vi "Create_Raw_data_file.vi"(4 "No of averages":i32=1, 5 "End time":dbl, 6 "Start time":dbl, 7 "Setup filename":string) -> (0 "Error String":string, 1 "Values":string[][](array[string]), 2 "Header Comments":string[](array[string]), 3 "Column headers":string[](array[string]))   [LabVIEW 2017]
uses:
  File/Setup_Filetype.ctl
  Controls/Post_Process.ctl
  Globals/Preference_global.vi
  Globals/Meas_global.vi
  Globals/Trav_pos_global.vi
  Globals/Constants_global.vi
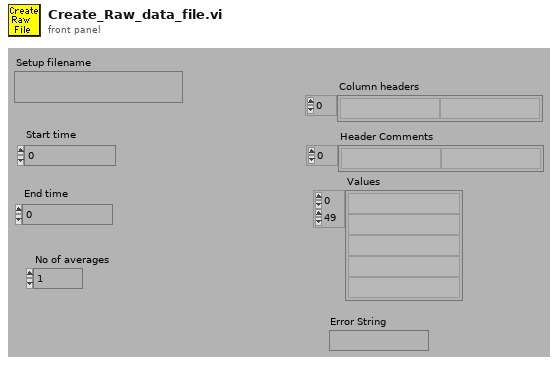
[diagram p1: front panel]
types:
  T1 = typedef "Post_Process.ctl" = enum16{"Take New Data", "Post Process Raw Data File"}
  T2 = typedef "Server_Comms.ctl" = enum16{"Server Link Healthy", "Do Not Link To Server"}
  T3 = typedef "Setup_Filetype.ctl" = enum16{"Measurement Setups", "Calibration Setups", "General", "Results File Plotter Setups", "Speed Calib Tweaks"}
  T4 = typedef "Traverse_cluster.ctl" = cluster{"Start X":sgl, "Start Y":sgl, "Start Z":sgl, "End X":sgl, "End Y":sgl, "End Z":sgl, "No. of pts.":i32, "Spacing":T5, "Filename":path, "Tunnel Speed":dbl, "Averaging time (min)":dbl, "Extra Commands":string, "Carrier_1 Q (l/min)":dbl, "Carrier_2 Q (l/min)":dbl, "Trace Gas Concentration (%)":dbl, "Specific Arguments":string, "Comments":string, "Row No":i32, "Row Type Selector":T6, "Completion time":string, "Row Duration (mins)":dbl, "No. of Valid pts.":i32, "Meas Setup File":string}
  T5 = typedef "Spacing.ctl" = enum16{"Linear", "Log", "Gauss", "Specified", "N/A"}
  T6 = typedef "Multi_run_mode.ctl" = enum16{"Move Traverse Only", "Set Tunnel Speed Only", "Set Source Only", "Set Measurement Conditions", "Single Measurement", "Vertical Profile", "Lateral Profile", "Longitudinal Profile", "Explore Volume", "Multi-Axis Profile", "Auto Calibrate", "Meas Fast FID Bkgnd", "Check Beam Power", "Scanning Valve Measurement", "Run VI Named:", "Set ADAM Ch", "Wait (minutes)", "Send Message", "Synchronize With:", "Fall Back to this Row", "Turn Off Row Repeating", "Blank Row", "Traverse 3D Volume"}
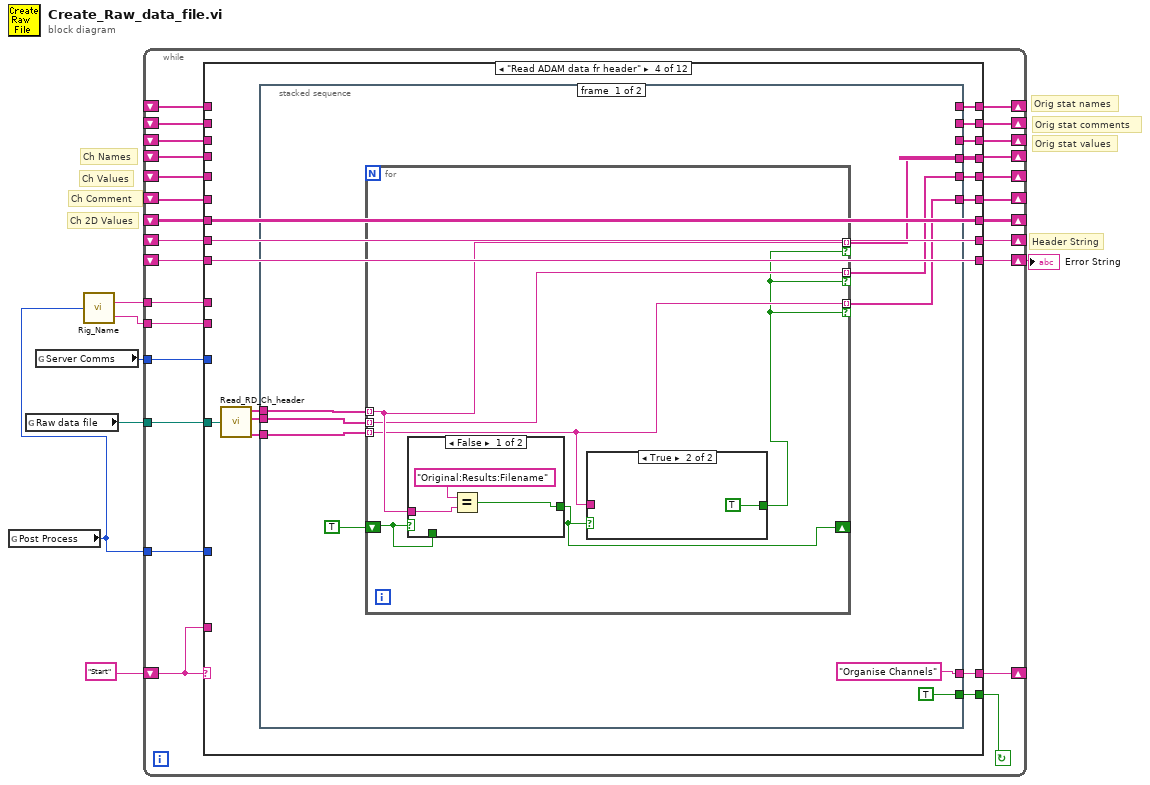
[diagram p0: block diagram]
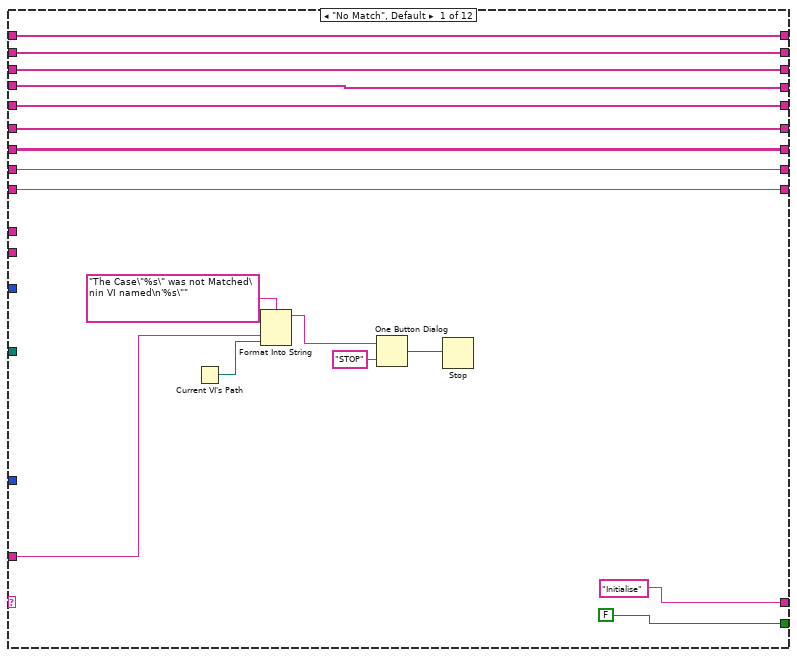
[diagram p2: hidden frame]
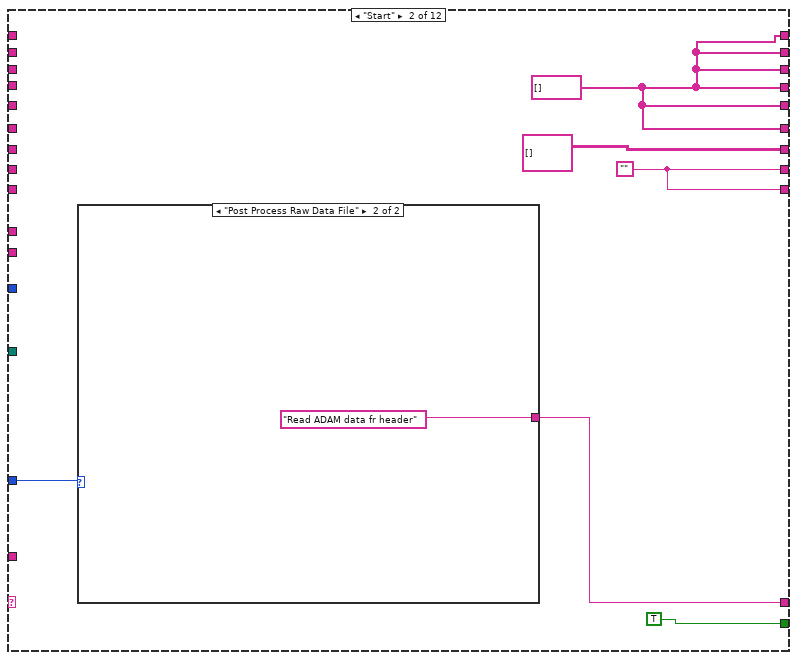
[diagram p3: hidden frame]
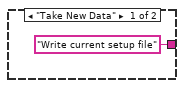
[diagram p4: hidden frame]
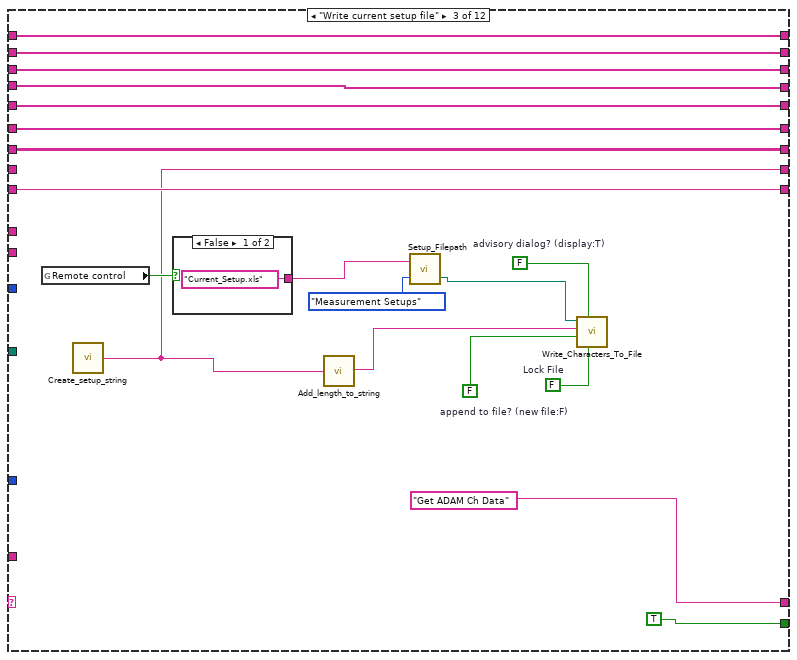
[diagram p5: hidden frame]
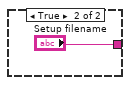
[diagram p6: hidden frame]
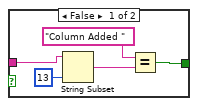
[diagram p7: hidden frame]
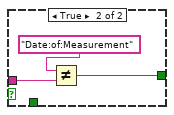
[diagram p8: hidden frame]
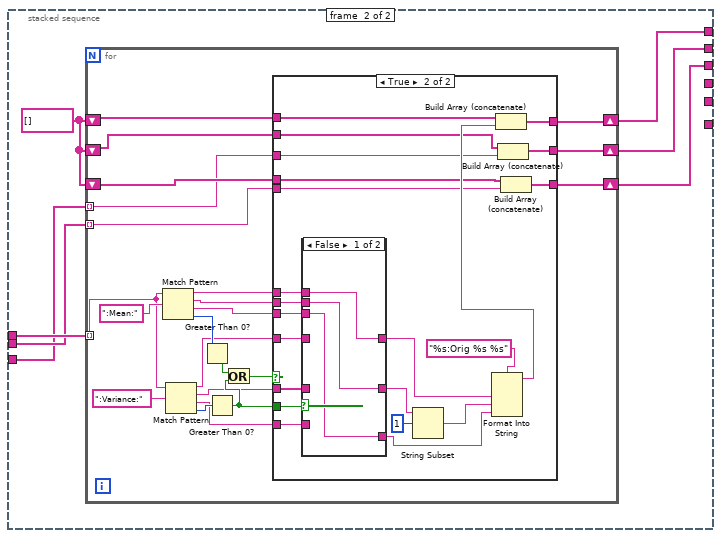
[diagram p9: hidden frame]
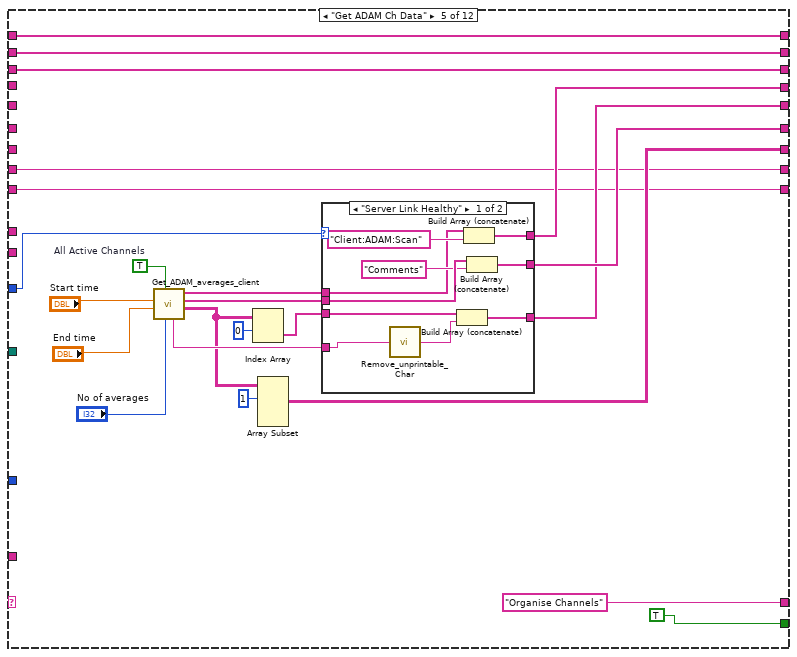
[diagram p12: hidden frame]
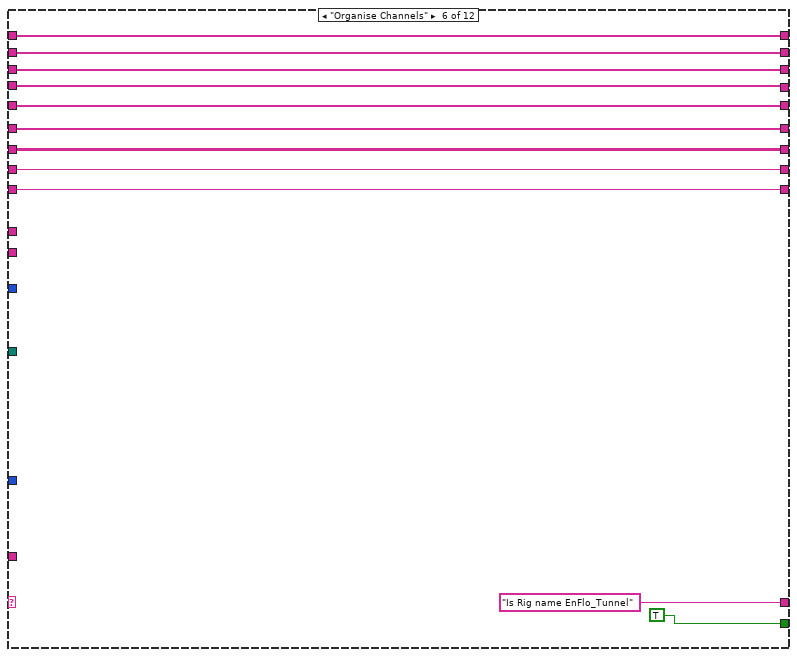
[diagram p14: hidden frame]
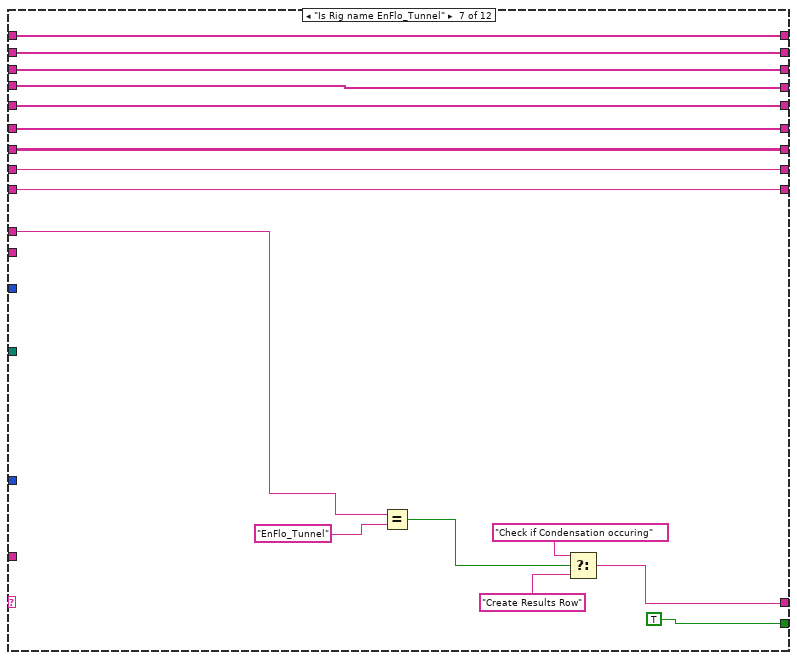
[diagram p15: hidden frame]
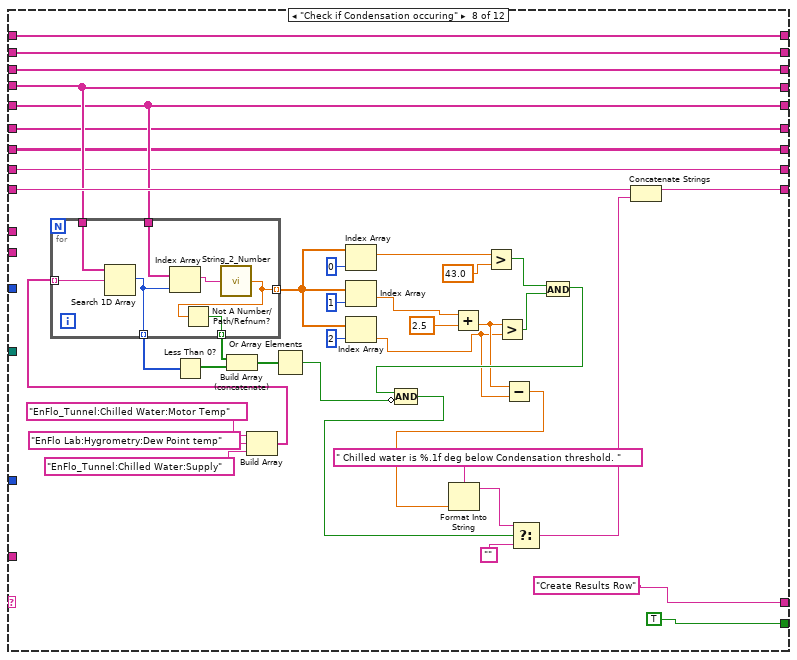
[diagram p16: hidden frame]
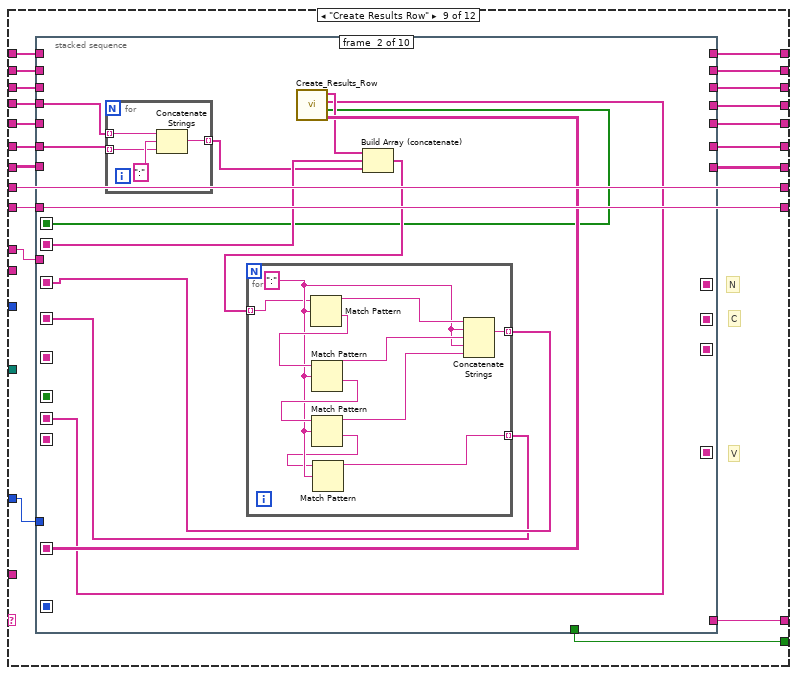
[diagram p17: hidden frame]
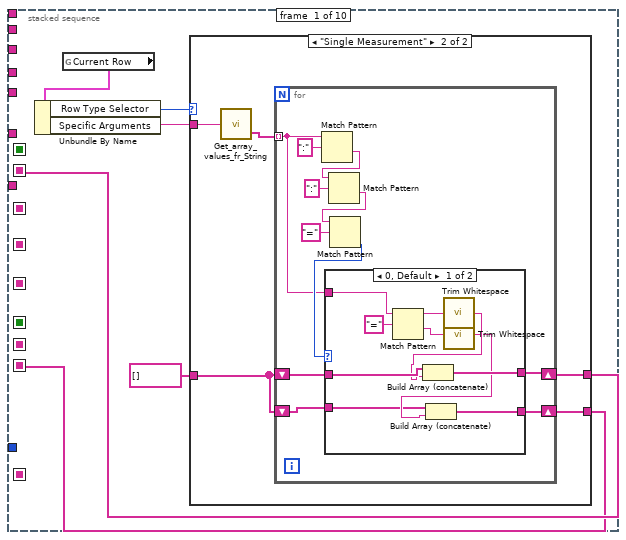
[diagram p18: hidden frame]
diagram:
  # "Orig stat values"
  # "Orig stat comments"
  # "Orig stat names"
  # "Header String"
  # "Ch 2D Values"
  # "Ch Comment"
  # "Ch Values"
  # "Ch Names"
  n1 = global read "Meas_global.vi" "Post Process"() -> (w3:T1)
  n2 = global read "Meas_global.vi" "Raw data file"() -> (w6:path)
  n3 = global read "Preference_global.vi" "Server Comms"() -> (w5:T2)
  n4 = call "Rig_Name.vi"("Post Process"=w3) -> ("Rig Setup before dash"=w2:string, "Hard Disk name"=w1:string)
  n5 = while {
    tunnel: w5 -> [w16]
    tunnel: w6 -> [w17]
    tunnel: w3 -> [w18]
    shift-left: _ -> [w20]
    shift-right: [w19] -> _
    shift-left: _ -> [w26]
    shift-right: [w25] -> w4
    shift-left: _ -> [w21]
    shift-right: [w27] -> _
    shift-left: _ -> [w22]
    shift-right: [w29] -> _
    shift-left: _ -> [w23]
    shift-right: [w28] -> _
    shift-left: _ -> [w24]
    shift-right: [w30] -> _
    shift-left: "Start" -> [w31]
    shift-right: [w32] -> _
    tunnel: w2 -> [w15]
    tunnel: w1 -> [w14]
    shift-right: [w10] -> _
    shift-left: _ -> [w11]
    shift-right: [w8] -> _
    shift-left: _ -> [w9]
    shift-right: [w12] -> _
    shift-left: _ -> [w13]
    stop <- w33 continue-if-true
    n6 = case shown="\"Read ADAM data fr header\"" w31 {
      tunnel: [FALSE TRUE TRUE w83 TRUE TRUE TRUE TRUE w299 TRUE TRUE FALSE] -> w33
      tunnel: ["Initialise" w52 "Get ADAM Ch Data" w94 "Organise Channels" "Is Rig name EnFlo_Tunnel" w236 "Create Results Row" w311 "Add Raw Data header info" "Add Raw Data fr Tempory file" "End"] -> w32
      tunnel: w31 -> [w45 _ _ _ _ _ _ _ _ _ _ _]
      tunnel: [w42 w51 w77 w85 w192 w226 w244 w254 w308 w614 w644 w661] -> w30
      tunnel: [w40 w51 w75 w86 w191 w224 w242 w252 w305 w625 w646 w663] -> w29
      tunnel: [w41 w51 w76 w84 w190 w225 w243 w253 w301 w626 w645 w662] -> w28
      tunnel: [w39 string[][] [] w74 w92 w188 w223 w241 w251 w303 w617 w647 w664] -> w27
      tunnel: w26 -> [w38 _ w72 w93 w187 w221 w238 w257 w309 w630 w648 w665]
      tunnel: [w38 w54 w72 w93 w187 w221 w238 w255 w309 w630 w648 w665] -> w25
      tunnel: w24 -> [w42 _ w77 _ _ w226 w244 w254 w307 w614 w644 w661]
      tunnel: w23 -> [w41 _ w76 _ _ w225 w243 w253 w302 w626 w645 w662]
      tunnel: w22 -> [w40 _ w75 _ _ w224 w242 w252 w306 w625 w646 w663]
      tunnel: w21 -> [w39 _ w74 w92 _ w223 w241 w251 w304 w617 w647 w664]
      tunnel: w20 -> [w37 _ _ w91 w186 w222 w239 w249 w310 w619 w641 w660]
      tunnel: [w37 w54 w66 w91 w186 w222 w239 w249 w310 w622 w640 ""] -> w19
      tunnel: w18 -> [_ w53 _ _ _ _ _ _ w300 _ _ _]
      tunnel: w17 -> [_ _ _ w90 _ _ _ _ _ _ _ w656]
      tunnel: w16 -> [_ _ _ _ w185 _ _ _ _ _ _ _]
      tunnel: w15 -> [_ _ _ _ _ _ w233 _ w298 _ _ _]
      tunnel: w14 -> [_ _ _ _ _ _ _ _ _ _ _ _]
      tunnel: w13 -> [w36 _ w64 _ w184 w220 w231 w248 w296 w611 w639 w653]
      tunnel: [w36 w51 w64 w82 w184 w220 w231 w248 w297 w611 w639 w653] -> w12
      tunnel: w11 -> [w35 _ w63 _ w183 w219 w230 w247 w295 w610 w638 w652]
      tunnel: [w35 w51 w63 w81 w183 w219 w230 w247 w294 w610 w638 w652] -> w10
      tunnel: w9 -> [w34 _ w62 _ w182 w218 w229 w246 w292 w609 w637 w651]
      tunnel: [w34 w51 w62 w80 w182 w218 w229 w246 w293 w609 w637 w651] -> w8
      frame "No Match", Default {
        n7 = Current VI's Path() -> (path=w44:path)
        n8 = Format Into String(format string="The Case\"%s\" was not Matched\nin VI named\n'%s\"" ("Format String"), w45, w44) -> (resulting string=w48:string)  [unwired: 2 in, 1 out]
        n9 = One Button Dialog(message=w48, button name ("OK")="STOP") -> (true=w46:bool)
        n10 = Stop(stop? (T)=w46) -> ()
      }
      frame "Start" {
        w54 = ""
        w51 = string[] []
        n11 = case shown="\"Post Process Raw Data File\"" w53 {
          tunnel: ["Write current setup file" "Read ADAM data fr header"] -> w52
          frame "Take New Data" {
          }
          frame "Post Process Raw Data File" {
          }
        }
      }
      frame "Write current setup file" {
        w67 = FALSE  # Lock File
        w70 = FALSE  # advisory dialog? (display:T)
        w71 = FALSE  # append to file? (new file:F)
        n12 = global read "Meas_global.vi" "Remote control"() -> (w69:bool)
        n13 = call "Create_setup_string.vi"() -> ("Setup String"=w66:string)  [unwired: 1 out]
        n14 = case shown="False" w69 {
          tunnel: ["Current_Setup.xls" ("Setup filename") "Setup filename"] -> w60
          frame False {
          }
          frame True {
          }
        }
        n15 = call "Add_length_to_string.vi"("String in"=w66) -> ("String out"=w68:string)
        n16 = call "Setup_Filepath.vi"("Setup File Type"=Setup_Filetype."Measurement Setups", "Filename in"=w60) -> ("Filename Out"=w59:path)  [unwired: 1 out]
        n17 = call "Write_Characters_To_File.vi"("file path (dialog if empty)"=w59, "advisory dialog? (display:T)"=w70, "character string"=w68, "append to file? (new file:F)"=w71, "Lock File"=w67) -> ()  [unwired: 4 out]
      }
      frame "Read ADAM data fr header" {
        n18 = call "Read_RD_Ch_header.vi"("Raw data file"=w90) -> ("Ch Name Out"=w88:string[], "Ch Values"=w87:string[], "Comments"=w89:string[])  [unwired: 1 out]
        n19 = stacked-sequence {
          tunnel: ["Organise Channels" _] -> w94
          tunnel: w89 -> [w101 w125]
          tunnel: w88 -> [w100 w128]
          tunnel: w87 -> [w99 w126]
          tunnel: [w95 _] -> w86
          tunnel: [w97 _] -> w85
          tunnel: [w96 _] -> w84
          tunnel: [TRUE _] -> w83
          tunnel: [_ w124] -> w82
          tunnel: [_ w123] -> w81
          tunnel: [_ w122] -> w80
          frame #0 {
            n20 = for {
              shift-right: [w108] -> _
              shift-left: TRUE -> [w109]
              tunnel: w100 -> [w107] mode=indexing
              tunnel: w101 -> [w105] mode=indexing
              tunnel: w99 -> [w106] mode=indexing
              tunnel: [w107] -> w97 mode=indexing if=w104
              tunnel: [w106] -> w96 mode=indexing if=w104
              tunnel: [w105] -> w95 mode=indexing if=w104
              n21 = case shown="False" w109 {
                tunnel: w107 -> [w117 w121]
                tunnel: [w116 w119] -> w108
                tunnel: w109 -> [_ _]
                frame False {
                  n22 = Equal?(x="Original:Results:Filename", y=w117) -> (x = y?=w116:bool)
                }
                frame True {
                  n23 = Not Equal?(x="Date:of:Measurement", y=w121) -> (x != y?=w119:bool)
                }
              }
              n24 = case shown="True" w108 {
                tunnel: w105 -> [w111 _]
                tunnel: [w113 TRUE] -> w104
                frame False {
                  n25 = String Subset(string=w111, length (rest)=13 ("length (rest)")) -> (substring=w110:string)  [unwired: 1 out]
                  n26 = Equal?(x="Column Added ", y=w110) -> (x = y?=w113:bool)
                }
                frame True {
                }
              }
            }
          }
          frame #1 {
            w127 = string[] []
            n27 = for {
              shift-right: [w136] -> w124
              shift-left: w127 -> [w135]
              shift-right: [w129] -> w123
              shift-left: w127 -> [w130]
              shift-right: [w132] -> w122
              shift-left: w127 -> [w133]
              tunnel: w128 -> [w148] mode=indexing
              tunnel: w126 -> [w134] mode=indexing
              tunnel: w125 -> [w131] mode=indexing
              n28 = Match Pattern(string=w148, regular expression=":Mean:") -> (before substring=w139:string, match substring=w138:string, after substring=w137:string, offset past match=w147:i32)  [unwired: 1 out]
              n29 = Match Pattern(string=w148, regular expression=":Variance:") -> (before substring=w142:string, match substring=w141:string, after substring=w140:string, offset past match=w146:i32)  [unwired: 1 out]
              n30 = Greater Than 0?(x=w147) -> (x > 0?=w145:bool)
              n31 = Greater Than 0?(x=w146) -> (x > 0?=w143:bool)
              n32 = Or(x=w145, y=w143) -> (x .or. y?=w144:bool)
              n33 = case shown="True" w144 {
                tunnel: w143 -> [_ w175]
                tunnel: w142 -> [_ w174]
                tunnel: w141 -> [_ w173]
                tunnel: w140 -> [_ w172]
                tunnel: w139 -> [_ w165]
                tunnel: w138 -> [_ w164]
                tunnel: w137 -> [_ w163]
                tunnel: [w153 w161] -> w136
                tunnel: w135 -> [w153 w160]
                tunnel: w134 -> [_ w159]
                tunnel: w133 -> [w151 w158]
                tunnel: [w151 w157] -> w132
                tunnel: w131 -> [_ w156]
                tunnel: w130 -> [w152 w155]
                tunnel: [w152 w154] -> w129
                frame False {
                }
                frame True {
                  n34 = case shown="False" w175 {
                    tunnel: w174 -> [_ w180]
                    tunnel: w173 -> [_ w181]
                    tunnel: w172 -> [_ w179]
                    tunnel: [w177 w181] -> w170
                    tunnel: [w178 w180] -> w167
                    tunnel: [w176 w179] -> w166
                    tunnel: w165 -> [w178 _]
                    tunnel: w164 -> [w177 _]
                    tunnel: w163 -> [w176 _]
                    frame False {
                    }
                    frame True {
                    }
                  }
                  n35 = String Subset(string=w170, offset (0)=1) -> (substring=w169:string)  [unwired: 1 out]
                  n36 = Format Into String(format string="%s:Orig %s %s", w167, w169, w166) -> (resulting string=w162:string)  [unwired: 2 in, 1 out]
                  n37 = Build Array (concatenate)(w160, w162) -> (w161:string[])
                  n38 = Build Array (concatenate)(w155, w156) -> (w154:string[])
                  n39 = Build Array (concatenate)(w158, w159) -> (w157:string[])
                }
              }
            }
          }
        }
      }
      frame "Get ADAM Ch Data" {
        w195 = TRUE  # All Active Channels
        n40 = call "Get_ADAM_averages_client.vi"("No of averages"="No of averages", "All Active Channels"=w195, "End time"="End time", "Start time"="Start time") -> ("Values"=w198:string[][], "Comments"=w201:string[], "Titles"=w200:string[], "Messages"=w202:string)  [unwired: 1 in, 3 out]
        n41 = Index Array(array=w198, index (row)=0 ("Index")) -> (element=w189:string[])  [unwired: 1 in]
        n42 = Array Subset(array=w198, index (row)=1 ("Array Index")) -> (w188:string[][])  [unwired: 3 in]
        n43 = case shown="\"Server Link Healthy\"" w185 {
          tunnel: w202 -> [w206 _]
          tunnel: w201 -> [w214 w216]
          tunnel: w200 -> [w211 w217]
          tunnel: [w210 w217] -> w192
          tunnel: [w209 w216] -> w191
          tunnel: [w208 w215] -> w190
          tunnel: w189 -> [w207 w215]
          frame "Server Link Healthy" {
            n44 = call "Remove_unprintable_Char.vi"("Input String"=w206) -> ("Output String"=w205:string)
            n45 = Build Array (concatenate)(w207, w205) -> (w208:string[])
            n46 = Build Array (concatenate)(w211, "Client:ADAM:Scan") -> (w210:string[])
            n47 = Build Array (concatenate)(w214, "Comments" ("Comments")) -> (w209:string[])
          }
          frame "Do Not Link To Server" {
          }
        }
      }
      frame "Organise Channels" {
      }
      frame "Is Rig name EnFlo_Tunnel" {
        n48 = Equal?(x=w233, y="EnFlo_Tunnel") -> (x = y?=w237:bool)
        n49 = Select(t="Check if Condensation occuring", s=w237, f="Create Results Row") -> (s? t:f=w236:string)
      }
      frame "Check if Condensation occuring" {
        n50 = Build Array("EnFlo_Tunnel:Chilled Water:Motor Temp", "EnFlo Lab:Hygrometry:Dew Point temp", "EnFlo_Tunnel:Chilled Water:Supply") -> (w280:string[])
        n51 = for {
          tunnel: w254 -> [w291]
          tunnel: w280 -> [w290] mode=indexing
          tunnel: w253 -> [w289]
          tunnel: [w287] -> w281 mode=indexing
          tunnel: [w286] -> w279 mode=indexing
          tunnel: [w285] -> w272 mode=indexing
          n52 = Search 1D Array(1D array=w291, element=w290) -> (index of element=w287:i32)  [unwired: 1 out]
          n53 = Index Array(array=w289, index=w287) -> (element=w288:string)
          n54 = call "String_2_Number.vi"("Value"=w288) -> ("Numeric"=w286:dbl)
          n55 = Not A Number/Path/Refnum?(number/path/refnum=w286) -> (NaN/Path/Refnum?=w285:bool)
        }
        n56 = Less Than 0?(x=w281) -> (x < 0?=w271:bool[])
        n57 = Build Array (concatenate)(w272, w271) -> (w270:bool[])
        n58 = Or Array Elements(Boolean array=w270) -> (logical OR=w266:bool)
        n59 = Index Array(array=w279, index=0 ("Index")) -> (element=w273:dbl)
        n60 = Index Array(array=w279, index=1 ("Index")) -> (element=w269:dbl)
        n61 = Index Array(array=w279, index=2 ("Index")) -> (element=w261:dbl)
        n62 = Add(x=w269, y=2.5) -> (x+y=w262:dbl)
        n63 = Greater?(x=w273, y=43.0) -> (0:w267:bool)
        n64 = Greater?(x=w262, y=w261) -> (0:w268:bool)
        n65 = Subtract(x=w262, y=w261) -> (x-y=w260:dbl)
        n66 = Format Into String(format string=" Chilled water is %.1f deg below Condensation threshold. " ("Format String"), w260) -> (resulting string=w258:string)  [unwired: 2 in, 1 out]
        n67 = And(x=w267, y=w268) -> (x .and. y?=w265:bool)
        n68 = Compound Arithmetic op=AND(w265, invert w266) -> (w264:bool)
        n69 = Select(t=w258, s=w264, f="") -> (s? t:f=w256:string)
        n70 = Concatenate Strings(w257, w256) -> (w255:string)
      }
      frame "Create Results Row" {
        # "V"
        # "C"
        # "N"
        n71 = stacked-sequence {
          seq-local: [_ w350 _ _ _ _ _ _ _ _] -> [_ _ _ w392 w433 _ _ _ _ _]
          seq-local: [_ w349 _ _ _ _ _ _ _ _] -> [_ _ _ w388 w432 _ _ _ _ _]
          seq-local: [_ _ w372 _ _ _ _ _ _ _] -> [_ _ _ w386 w431 _ _ _ _ _]
          seq-local: [_ w357 _ _ _ _ _ _ _ _] -> [_ _ _ _ _ w469 _ _ _ _]
          seq-local: [_ _ _ _ w430 _ _ _ _ _] -> [_ _ _ _ _ w471 _ _ _ _]
          seq-local: [w313 _ _ _ _ _ _ _ _ _] -> [_ w353 _ _ _ _ _ _ _ _]
          seq-local: [w312 _ _ _ _ _ _ _ _ _] -> [_ _ w374 _ _ _ _ _ _ _]
          seq-local: [_ _ _ _ w429 _ _ _ _ _] -> [_ _ _ _ _ _ _ w542 w580 _]
          seq-local: [_ _ _ _ w428 _ _ _ _ _] -> [_ _ _ _ _ _ _ _ w578 _]
          seq-local: [_ _ _ _ _ w468 _ _ _ _] -> [_ _ _ _ _ _ _ _ w577 _]
          seq-local: [_ _ _ _ _ _ w502 _ _ _] -> [_ _ _ _ _ _ _ w541 w581 _]
          seq-local: [_ _ _ _ _ _ _ w540 _ _] -> [_ _ _ _ _ _ _ _ w579 _]
          seq-local: [_ w348 _ _ _ _ _ _ _ _] -> [_ _ w373 _ _ _ _ _ _ _]
          seq-local: [_ w347 _ _ _ _ _ _ _ _] -> [_ _ _ _ _ w467 _ _ _ _]
          tunnel: [_ _ "Add Adam Chs to header" _ _ _ _ _ _ _] -> w311
          tunnel: w307 -> [_ w356 _ w390 _ _ w505 _ _ _]
          tunnel: w306 -> [_ w355 _ w391 _ _ _ _ _ _]
          tunnel: w309 -> [_ _ w377 _ _ _ _ _ _ _]
          tunnel: w302 -> [_ _ w376 w385 _ _ w504 _ _ _]
          tunnel: w304 -> [_ _ w375 _ _ _ _ _ _ _]
          tunnel: [_ _ _ w389 _ _ _ _ _ _] -> w308
          tunnel: [_ _ _ w387 _ _ _ _ _ _] -> w305
          tunnel: [_ _ w375 _ _ _ _ _ _ _] -> w303
          tunnel: [_ _ _ w384 _ _ _ _ _ _] -> w301
          tunnel: w300 -> [_ _ _ w383 w434 _ w512 _ _ _]
          tunnel: [_ _ _ _ _ _ w508 _ _ _] -> w299
          tunnel: w298 -> [_ _ _ _ _ _ w506 _ _ _]
          tunnel: [_ _ _ _ _ _ _ _ _ w608] -> w297
          tunnel: w296 -> [_ _ _ _ _ _ _ _ w575 w608]
          tunnel: w295 -> [_ _ _ _ _ _ _ _ w572 w607]
          tunnel: [_ _ _ _ _ _ _ _ _ w607] -> w294
          tunnel: [_ _ _ _ _ _ _ _ _ w606] -> w293
          tunnel: w292 -> [_ _ _ _ _ _ _ _ w569 w606]
          frame #0 {
            n72 = global read "Trav_pos_global.vi" "Current Row"() -> (w317:T4)
            n73 = Unbundle By Name(w317) -> ("Row Type Selector"=w316:T6, "Specific Arguments"=w315:string)
            n74 = case shown="\"Single Measurement\"" w316 {
              tunnel: w315 -> [_ w323]
              tunnel: string[] [] -> [w318 w321]
              tunnel: [w318 w320] -> w313
              tunnel: [w318 w319] -> w312
              frame "Move Traverse Only", Default {
              }
              frame "Single Measurement" {
                n75 = call "Get_array_values_fr_String.vi"("String Value"=w323) -> ("String array"=w322:string[])  [unwired: 1 out]
                n76 = for {
                  tunnel: w322 -> [w326] mode=indexing
                  shift-right: [w324] -> w319
                  shift-left: w321 -> [w325]
                  shift-right: [w327] -> w320
                  shift-left: w321 -> [w328]
                  n77 = Match Pattern(string=w326, regular expression=":") -> (after substring=w332:string)  [unwired: 4 out]
                  n78 = Match Pattern(string=w332, regular expression=":") -> (after substring=w330:string)  [unwired: 4 out]
                  n79 = Match Pattern(string=w330, regular expression="=") -> (offset past match=w329:i32)  [unwired: 4 out]
                  n80 = case shown="0, Default" w329 {
                    tunnel: w328 -> [w344 w346]
                    tunnel: [w343 w346] -> w327
                    tunnel: w326 -> [w339 _]
                    tunnel: w325 -> [w336 w345]
                    tunnel: [w335 w345] -> w324
                    frame 0, Default {
                      n81 = Match Pattern(string=w339, regular expression="=") -> (before substring=w341:string, after substring=w340:string)  [unwired: 3 out]
                      n82 = call <vilib>:"Trim Whitespace.vi"("string"=w341) -> ("trimmed string"=w338:string)  [unwired: 1 in]
                      n83 = Build Array (concatenate)(w344, w338) -> (w343:string[])
                      n84 = call <vilib>:"Trim Whitespace.vi"("string"=w340) -> ("trimmed string"=w337:string)  [unwired: 1 in]
                      n85 = Build Array (concatenate)(w336, w337) -> (w335:string[])
                    }
                    frame -1 {
                    }
                  }
                }
              }
            }
          }
          frame #1 {
            n86 = for {
              tunnel: w356 -> [w370] mode=indexing
              tunnel: w355 -> [w369] mode=indexing
              tunnel: [w368] -> w352 mode=indexing
              n87 = Concatenate Strings(w370, ":" ("Substring"), w369) -> (w368:string)
            }
            n88 = call "Create_Results_Row.vi"() -> ("row splitting"=w357:string[][], "Values to Keep in Dup rows"=w347:bool[], "Channel Values"=w348:string[], "Channel Names"=w354:string[])  [unwired: 5 in]
            n89 = Build Array (concatenate)(w354, w353, w352) -> (w351:string[])
            n90 = for {
              tunnel: w351 -> [w358] mode=indexing
              tunnel: [w362] -> w350 mode=indexing
              tunnel: [w359] -> w349 mode=indexing
              w361 = ":" ("regular expression")
              n91 = Match Pattern(string=w358, regular expression=w361) -> (before substring=w365:string, after substring=w367:string)  [unwired: 3 out]
              n92 = Match Pattern(string=w367, regular expression=w361) -> (before substring=w364:string, after substring=w366:string)  [unwired: 3 out]
              n93 = Match Pattern(string=w366, regular expression=w361) -> (before substring=w363:string, after substring=w360:string)  [unwired: 3 out]
              n94 = Match Pattern(string=w360, regular expression=w361) -> (before substring=w359:string)  [unwired: 4 out]
              n95 = Concatenate Strings(w365, w361, w364, w361, w363) -> (w362:string)
            }
          }
          frame #2 {
            w378 = 5  # Comment Column
            n96 = Index Array(array=w373, index=w378) -> (element=w380:string)
            n97 = Concatenate Strings(w380, w377) -> (w381:string)
            n98 = Replace Array Subset(array=w373, new element=w381, index=w378) -> (w379:string[])
            n99 = Build Array (concatenate)(w379, w374, w376) -> (w372:string[])
          }
          frame #3 {
            n100 = case shown="\"Post Process Raw Data File\"" w383 {
              tunnel: w392 -> [w401 _]
              tunnel: w391 -> [w400 w426]
              tunnel: w390 -> [w399 w427]
              tunnel: [w398 w427] -> w389
              tunnel: w388 -> [w397 _]
              tunnel: [w396 w426] -> w387
              tunnel: w386 -> [w395 _]
              tunnel: w385 -> [w394 w425]
              tunnel: [w393 w425] -> w384
              frame "Take New Data" {
                n101 = for {
                  tunnel: w399 -> [w412]
                  tunnel: w401 -> [w408] mode=indexing
                  shift-right: [w409] -> w398
                  shift-left: w399 -> [w410]
                  shift-right: [w406] -> w396
                  shift-left: w400 -> [w407]
                  shift-right: [w403] -> w393
                  shift-left: w394 -> [w404]
                  tunnel: w397 -> [w405] mode=indexing
                  tunnel: w395 -> [w402] mode=indexing
                  n102 = Search 1D Array(1D array=w412, element=w408) -> (index of element=w411:i32)  [unwired: 1 out]
                  n103 = case shown="0, Default" w411 {
                    tunnel: w410 -> [w415 w424]
                    tunnel: [w415 w422] -> w409
                    tunnel: w408 -> [_ w423]
                    tunnel: w407 -> [w414 w421]
                    tunnel: [w414 w420] -> w406
                    tunnel: w405 -> [_ w419]
                    tunnel: w404 -> [w413 w417]
                    tunnel: [w413 w416] -> w403
                    tunnel: w402 -> [_ w418]
                    frame 0, Default {
                    }
                    frame -1 {
                      n104 = Build Array (concatenate)(w417, w418) -> (w416:string[])
                      n105 = Build Array (concatenate)(w424, w423) -> (w422:string[])
                      n106 = Build Array (concatenate)(w421, w419) -> (w420:string[])
                    }
                  }
                }
              }
              frame "Post Process Raw Data File" {
              }
            }
          }
          frame #4 {
            # "Values"
            # "Comments"
            # "Ch Names"
            n107 = case shown="\"Post Process Raw Data File\"" w434 {
              tunnel: [w437 w443] -> w429
              tunnel: w433 -> [w437 w444]
              tunnel: [w436 w442] -> w428
              tunnel: w432 -> [w436 w440]
              tunnel: [w435 w441] -> w430
              tunnel: w431 -> [w435 w439]
              frame "Take New Data" {
              }
              frame "Post Process Raw Data File" {
                w438 = string[] []
                n108 = for {
                  shift-right: [w452] -> w443
                  shift-left: w438 -> [w453]
                  shift-right: [w447] -> w442
                  shift-left: w438 -> [w450]
                  shift-right: [w448] -> w441
                  shift-left: w438 -> [w449]
                  tunnel: w444 -> [w451] mode=indexing
                  tunnel: w440 -> [w446] mode=indexing
                  tunnel: w439 -> [w445] mode=indexing
                  n109 = Search 1D Array(1D array=w453, element=w451) -> (index of element=w454:i32)  [unwired: 1 out]
                  n110 = case shown="-1" w454 {
                    tunnel: w453 -> [w457 w466]
                    tunnel: [w457 w465] -> w452
                    tunnel: w451 -> [_ w464]
                    tunnel: w450 -> [w456 w463]
                    tunnel: w449 -> [w455 w462]
                    tunnel: [w455 w461] -> w448
                    tunnel: [w456 w460] -> w447
                    tunnel: w446 -> [_ w459]
                    tunnel: w445 -> [_ w458]
                    frame 0, Default {
                    }
                    frame -1 {
                      n111 = Build Array (concatenate)(w466, w464) -> (w465:string[])
                      n112 = Build Array (concatenate)(w463, w459) -> (w460:string[])
                      n113 = Build Array (concatenate)(w462, w458) -> (w461:string[])
                    }
                  }
                }
              }
            }
          }
          frame #5 {
            n114 = Array Size(array=w469) -> (size(s)=w474:i32[])
            n115 = Index Array(array=w474, index=0) -> (element=w472:i32)
            n116 = Greater Than 0?(x=w472) -> (x > 0?=w470:bool)
            n117 = case shown="True" w470 {
              tunnel: w471 -> [w476 w482]
              tunnel: w469 -> [_ w484]
              tunnel: [w475 w483] -> w468
              tunnel: w467 -> [_ w478]
              frame False {
                n118 = Build Array(w476) -> (w475:string[][])
              }
              frame True {
                n119 = Array Size(array=w482) -> (size(s)=w481:i32)
                n120 = Search 1D Array(1D array=w482, element="Instrument_name_place_holder") -> (index of element=w485:i32)  [unwired: 1 out]
                n121 = Initialize Array(TRUE, w481) -> (w479:bool[])
                n122 = Build Array (concatenate)(w478, w479) -> (w477:bool[])
                n123 = for {
                  tunnel: w482 -> [w493]
                  tunnel: w485 -> [w492]
                  tunnel: w484 -> [w491] mode=indexing
                  tunnel: [w488] -> w483 mode=indexing
                  tunnel: w477 -> [w487]
                  i -> [w490]
                  n124 = Replace Array Subset(array=w493, new element=w491, index=w492) -> (w489:string[])
                  n125 = case shown="1, Default" w490 {
                    tunnel: w489 -> [w494 w496]
                    tunnel: [w494 w495] -> w488
                    tunnel: w487 -> [_ w497]
                    frame 0 {
                    }
                    frame 1, Default {
                      n126 = for {
                        tunnel: w497 -> [w501] mode=indexing
                        tunnel: w496 -> [w500] mode=indexing
                        tunnel: [w499] -> w495 mode=indexing
                        n127 = Select(t=w500, s=w501, f="") -> (s? t:f=w499:string)
                      }
                    }
                  }
                }
              }
            }
          }
          frame #6 {
            n128 = Equal?(x="EnFlo_Tunnel", y=w506) -> (x = y?=w503:bool)
            n129 = case shown="True" w503 {
              tunnel: w505 -> [_ w521]
              tunnel: w504 -> [_ w518]
              tunnel: [FALSE w516] -> w502
              frame False {
              }
              frame True {
                n130 = disable-structure shown="Enabled" {
                  disable-tunnel: [w522 FALSE] -> w514
                  frame Disabled {
                    n131 = global read "Meas_global.vi" "Pre Setup String"() -> (w526:string)
                    n132 = call "Get_Characters_from_string.vi"("Input string"=w526, "Variable name"="Show_all_EnFlo_Tunnel_Columns") -> ("Status"=w524:enum16{"Char in string", "Char not in string"}, "Value"=w523:string)  [unwired: 1 in]
                    n133 = case shown="\"Char in string\"" w524 {
                      tunnel: w523 -> [w529 _]
                      tunnel: [w527 TRUE] -> w522
                      frame "Char in string" {
                        n134 = Equal?(x=w529, y="TRUE") -> (x = y?=w528:bool)
                        n135 = Not(x=w528) -> (.not. x?=w527:bool)
                      }
                      frame "Char not in string" {
                      }
                    }
                  }
                  frame Enabled {
                  }
                }
                n136 = Search 1D Array(1D array=w521, element="EnFlo_Tunnel:Heater:Enable") -> (index of element=w519:i32)  [unwired: 1 out]
                n137 = case shown="-1" w519 {
                  tunnel: w519 -> [w538 _]
                  tunnel: w518 -> [w537 _]
                  tunnel: [w533 FALSE] -> w517
                  frame 0, Default {
                    n138 = Index Array(array=w537, index=w538) -> (element=w536:string)
                    n139 = call "String_2_Number.vi"("Value"=w536) -> ("Numeric"=w535:dbl)
                    n140 = Less?(x=w535, y=0.5) -> (x < y?=w533:bool)
                  }
                  frame -1 {
                  }
                }
                n141 = Select(t=w517, s=w514, f=FALSE) -> (s? t:f=w516:bool)
              }
            }
            n142 = global read "Trav_pos_global.vi" "Dummy Measurement?"() -> (w509:bool)
            n143 = Equal?(x=Post_Process."Take New Data" ("Post Process"), y=w512) -> (x = y?=w510:bool)
            n144 = Compound Arithmetic op=AND(invert w509, w510) -> (w508:bool)
          }
          frame #7 {
            n145 = case shown="True" w541 {
              tunnel: w542 -> [_ w548]
              tunnel: [i32[] [] w546] -> w540
              frame False {
              }
              frame True {
                w544 = string[] ["EnFlo_Tunnel:Inlet Heater:Temp", "EnFlo_Tunnel:Inlet Rake:Temp", "EnFlo_Tunnel:Trav Thermo:", "EnFlo_Tunnel:floor ", "EnFlo_Tunnel:roof ", "EnFlo_Tunnel:Side ", "EnFlo_Tunnel:Temp:Inlet", "EnFlo_Tunnel:Temp:Floor"] ("Column headers")
                # "Remove these\nChannels"
                # "Remaining\nChannels"
                n146 = for {
                  tunnel: w544 -> [w550] mode=indexing
                  tunnel: [w549] -> w545 mode=indexing
                  n147 = String Length(string=w550) -> (length=w549:i32)
                }
                n148 = for {
                  tunnel: w548 -> [w554] mode=indexing
                  shift-right: [w557] -> w546
                  shift-left: i32[] [] -> [w558]
                  tunnel: w545 -> [w555]
                  tunnel: w544 -> [w553]
                  i -> [w556]
                  n149 = for {
                    tunnel: w555 -> [w563] mode=indexing
                    tunnel: w554 -> [w562]
                    tunnel: w553 -> [w560] mode=indexing
                    tunnel: [w559] -> w552 mode=indexing
                    n150 = String Subset(string=w562, length (rest)=w563) -> (substring=w561:string)  [unwired: 1 out]
                    n151 = Equal?(x=w561, y=w560) -> (x = y?=w559:bool)
                  }
                  n152 = Or Array Elements(Boolean array=w552) -> (logical OR=w551:bool)
                  n153 = case shown="True" w551 {
                    tunnel: w558 -> [w566 w567]
                    tunnel: w556 -> [w565 _]
                    tunnel: [w564 w567] -> w557
                    frame False {
                      n154 = Build Array (concatenate)(w566, w565) -> (w564:i32[])
                    }
                    frame True {
                    }
                  }
                }
              }
            }
          }
          frame #8 {
            n155 = case shown="True" w581 {
              tunnel: w580 -> [w587 w594]
              tunnel: w579 -> [_ w589]
              tunnel: w578 -> [w586 w593]
              tunnel: [w587 w592] -> w576
              tunnel: [w586 w591] -> w573
              tunnel: w577 -> [w585 w590]
              tunnel: [w585 w588] -> w570
              frame False {
              }
              frame True {
                n156 = for {
                  tunnel: w590 -> [w597] mode=indexing
                  tunnel: w589 -> [w596]
                  tunnel: [w595] -> w588 mode=indexing
                  n157 = for {
                    tunnel: w597 -> [w599]
                    tunnel: w596 -> [w600] mode=indexing
                    tunnel: [w598] -> w595 mode=indexing
                    n158 = Index Array(array=w599, index=w600) -> (element=w598:string)
                  }
                }
                n159 = for {
                  tunnel: w594 -> [w605]
                  tunnel: w589 -> [w601] mode=indexing
                  tunnel: w593 -> [w604]
                  tunnel: [w603] -> w592 mode=indexing
                  tunnel: [w602] -> w591 mode=indexing
                  n160 = Index Array(array=w604, index=w601) -> (element=w602:string)
                  n161 = Index Array(array=w605, index=w601) -> (element=w603:string)
                }
              }
            }
            n162 = for {
              tunnel: w570 -> [w584] mode=indexing
              tunnel: w569 -> [w583]
              tunnel: [w582] -> w568 mode=indexing
              n163 = Build Array (concatenate)(w584, w583) -> (w582:string[])
            }
            "Values" <- w568
            n164 = Build Array (concatenate)(w576, w575) -> (→"Column headers":string[])
            n165 = Build Array (concatenate)(w573, w572) -> (→"Header Comments":string[])
          }
          frame #9 {
          }
        }
      }
      frame "Add Adam Chs to header" {
        w612 = FALSE  # Email On Error?
        n166 = call "Channel_name_checker.vi"("Email On Error?"=w612, "Channel names"=w614) -> ("Channel names Out"=w613:string[])  [unwired: 1 out]
        n167 = for {
          tunnel: w613 -> [w636] mode=indexing
          tunnel: [w635] -> w629 mode=indexing
          tunnel: [w634] -> w628 mode=indexing
          tunnel: [w633] -> w627 mode=indexing
          n168 = call "Split_Ch_name.vi"("Ch name"=w636) -> ("Top level"=w635:string, "Middle"=w634:string, "Low level"=w633:string)
        }
        n169 = Array To Spreadsheet String(array=w617, 3:"%s" ("format string")) -> (spreadsheet string=w615:string)  [unwired: 1 out]
        n170 = Build Array(w629, w628, w627, w626, w625) -> (w623:string[][])
        n171 = Array To Spreadsheet String(array=w623, 3:"%s" ("format string")) -> (spreadsheet string=w616:string)  [unwired: 1 out]
        n172 = Concatenate Strings(w616, w615, "***************************************" ("Substring"), "\r\n", w619) -> (w622:string)
      }
      frame "Add Raw Data header info" {
        n173 = String Length(string=w641) -> (length=w643:i32)
        n174 = call "Raw_Data_File_Start_text.vi"("Header length"=w643) -> ("Start String"=w642:string)
        n175 = Concatenate Strings(w642, w641) -> (w640:string)
      }
      frame "Add Raw Data fr Tempory file" {
        w654 = 0  # Start to copy file at:
        n176 = global read "Constants_global.vi" "Data Folder Local"() -> (w658:path)
        n177 = Build Path(base path=w658, name or relative path="Tempory_Raw_Data_File.xls") -> (appended path=w655:path)
        n178 = call "Piece_file_Copy.vi"("File Start String"=w660, "Start to copy file at:"=w654, "Source File"=w655, "Target File"=w656) -> ()  [unwired: 1 out]
      }
    }
  }
  "Error String" <- w4
